vi "MessageProbe.vi"(11 "Message":refnum<class "Message.lvclass">) -> (2 "Value String":string, 3 "Boolean":bool)   [LabVIEW 2018, in "LapDog.Messaging.v3.lvlib" / "Message.lvclass"]
uses:
  Message.lvclass
panel:
  out "Message Type":string
  out "Data":string
  out "Message Name":string
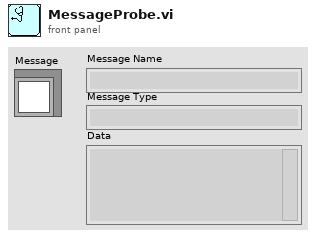
[diagram p1: front panel]
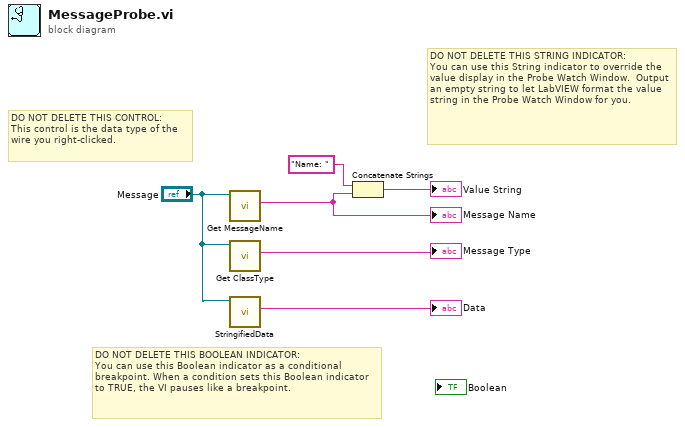
[diagram p0: block diagram]
diagram:
  # "DO NOT DELETE THIS STRING INDICATOR: \nYou can use this String indicator to override the value display in the Probe Watch Window.  Output an empty string to let LabVIEW format the value string in the Probe Watch Window for you."
  # "DO NOT DELETE THIS BOOLEAN INDICATOR: \nYou can use this Boolean indicator as a conditional breakpoint. When a condition sets this Boolean indicator to TRUE, the VI pauses like a breakpoint."
  # "DO NOT DELETE THIS CONTROL: \nThis control is the data type of the wire you right-clicked."
  n1 = call "Get MessageName.vi"("Message in"="Message") -> ("Message Name"=w1:string)  [unwired: 8 in, 2 out]
  "Message Name" <- w1
  n2 = call-dynamic "Get ClassType.vi"("Message in"="Message") -> ("Class Type"=→"Message Type":string)  [unwired: 8 in, 2 out]
  n3 = call-dynamic "StringifiedData.vi"("Message in"="Message") -> ("Stringified Data"=→"Data":string)  [unwired: 8 in, 2 out]
  n4 = Concatenate Strings("Name: " ("string"), w1) -> (→"Value String":string)
